vi "Init.vi"(8 "error in (no error)":errorcluster, 11 "Kasli Writer in":refnum<class "Kasli Writer.lvclass">) -> (0 "error out":errorcluster, 3 "Kasli Writer out":refnum<class "Kasli Writer.lvclass">)   [LabVIEW 2020, in "Kasli Listener and Writer.lvlib" / "Kasli Writer.lvclass"]
uses:
  Kasli Writer.lvclass
  Ancestor/Ancestor/Ancestor.lvclass
  Father of all uServices/Father of all uServices/Father of all uServices.lvclass
  C:/Users/marco/Documents/GitHub_Lab/TALOS/talos/Internal uServices/System uServices/TCP Writer/TCP Writer/TCP Writer.lvclass
  C:/Users/marco/Documents/GitHub_Lab/TALOS/talos/Father of all uServices/Father of all uServices/Father of all uServices.lvclass
  C:/Users/marco/Documents/GitHub_Lab/TALOS/talos/Ancestor/Ancestor/Ancestor.lvclass
  C:/Users/marco/Documents/GitHub_Lab/TALOS/builds/Actor Framework PPL/Actor Framework.lvlibp/1abvi3w/vi.lib/ActorFramework/Actor/Actor.lvclass
  System uServices/TCP Writer/TCP Writer/TCP Writer.lvclass
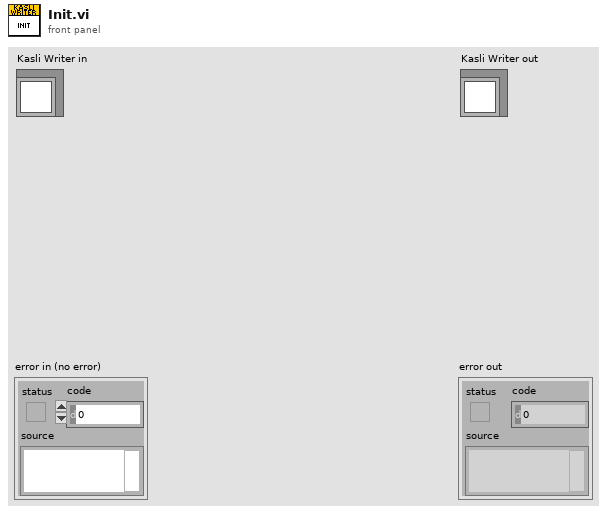
[diagram p1: front panel]
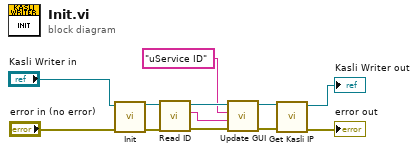
[diagram p0: block diagram]
diagram:
  n1 = call-parent "Init.vi"("error in (no error)"="error in (no error)", "TCP Writer in"="Kasli Writer in") -> ("error out"=w1:errorcluster, "TCP Writer out"=w2:refnum<class "Kasli Writer.lvclass">)  [unwired: 8 in]
  n2 = call "Read ID.vi"("error in (no error)"=w1, "Ancestor in"=w2) -> ("error out"=w8:errorcluster, "ID"=w5:string, "Ancestor out"=w7:refnum<class "Kasli Writer.lvclass">)  [unwired: 7 in]
  n3 = call "Update GUI.vi"("error in (no error)"=w8, "Data"=w5, "GUI Item Name"="uService ID", "uService Template in"=w7) -> ("error out"=w4:errorcluster, "uService Template out"=w3:refnum<class "Kasli Writer.lvclass">)  [unwired: 6 in]
  n4 = call-dynamic "Get Kasli IP.vi"("error in (no error)"=w4, "Kasli Writer in"=w3) -> ("error out"=→"error out":errorcluster, "Kasli Writer out"=→"Kasli Writer out":refnum<class "Kasli Writer.lvclass">)  [unwired: 8 in]
